vi "calibration setting.vi"() -> ()   [LabVIEW 2019, in "Calibration Lib.lvlib"]
uses:
  Calibration Lib.lvlib
  database.lvlib
panel:
  in  "Close":bool
  in  "Method 2 Verify":bool
  out "Error out":errorcluster
  in  "Calibration File Path":path
  out "Calibration String":string
  in  "Calibration Method":enum32{"Method 1", "Method 2"}(radio)=enum."Method 2"
  in  "Thresholds":bool
  in  "Method 2 Calibration":bool
  in  "Method 1 Calibration":bool
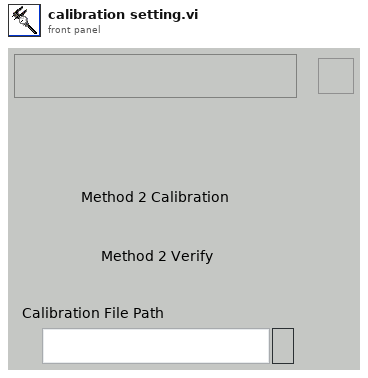
[diagram p1: front panel]
types:
  T1 = cluster{"Calibration Method":enum32{"Method 1", "Method 2"}, "Calibration File Path":path}
  T2 = enum8{"Enabled", "Disabled", "Disabled and Grayed Out"}
  T3 = cluster{"Calibration Method":u32, "Calibration File Path":path}[]
  T4 = cluster{"Calibration Method":u32, "Calibration File Path":path}
  T5 = cluster{"Calibration Method":enum32{"Method 1", "Method 2"}, string}
  T6 = cluster{i32, "date/time string":string, "date/time string":string, "table":string}
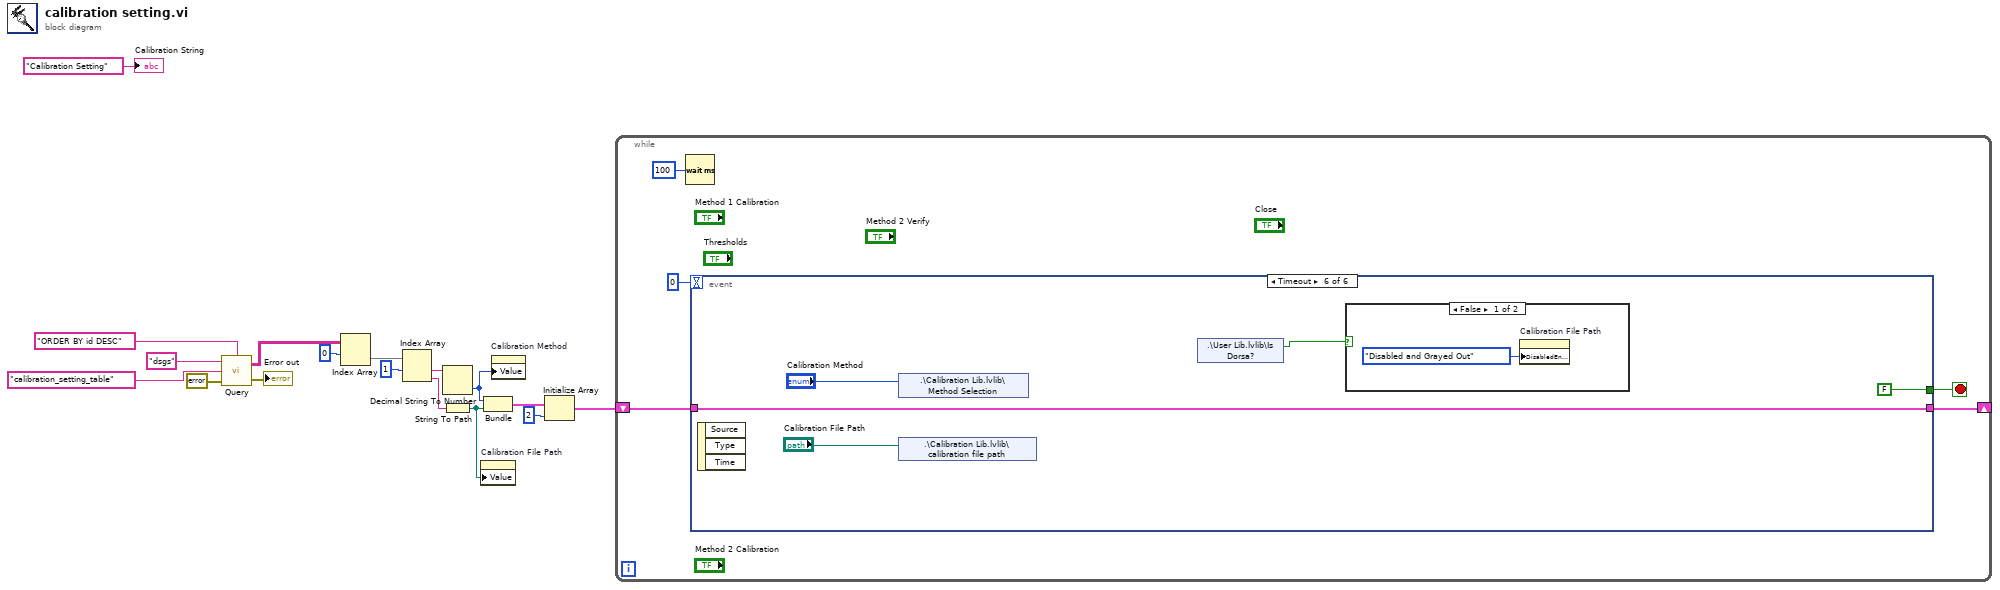
[diagram p0: block diagram]
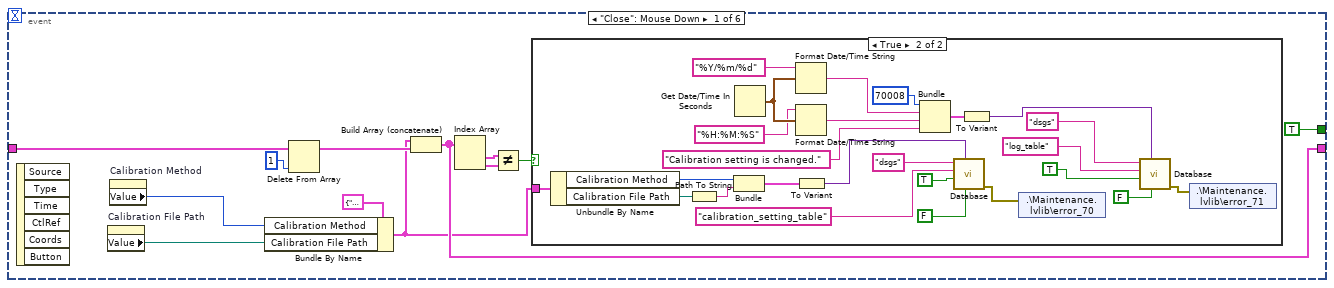
[diagram p2: hidden frame]
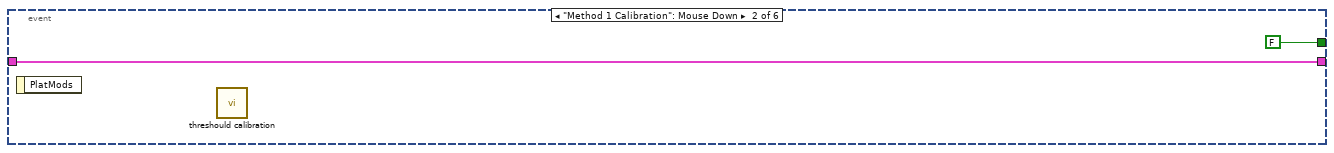
[diagram p4: hidden frame]
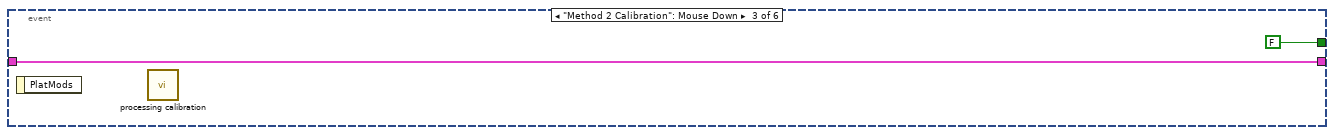
[diagram p5: hidden frame]
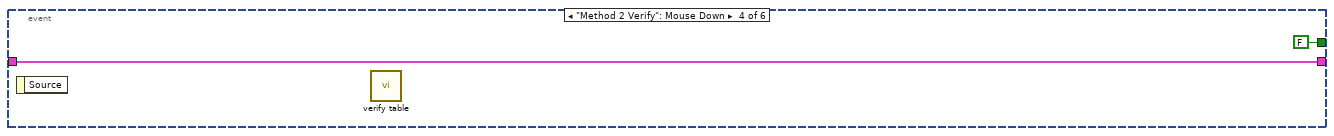
[diagram p6: hidden frame]
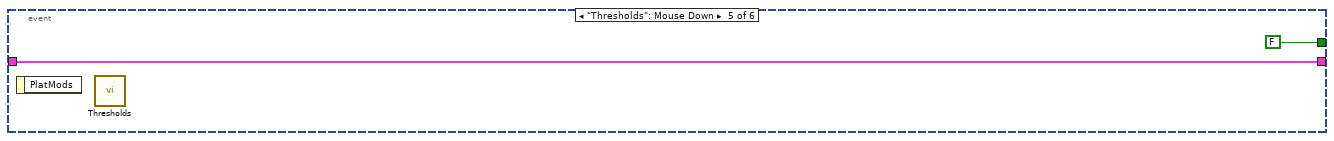
[diagram p7: hidden frame]
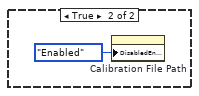
[diagram p8: hidden frame]
diagram:
  n1 = call "Query.vi"("Condition"="ORDER BY id DESC", "Error in"=errorcluster {"status"=FALSE, "code"=0, "source"=""}, "Table Name"="calibration_setting_table", "Connection Name"="dsgs") -> ("Error out"=→"Error out":errorcluster, "data"=w10:string[][])
  n2 = Index Array(array=w10, index (row)=0) -> (element=w8:string[])  [unwired: 1 in]
  n3 = Index Array(array=w8, index #1=1 ("index")) -> (element #1=w6:string, element #2=w4:string)  [unwired: 1 in]
  n4 = Decimal String To Number(string=w6) -> (number=w3:i32)  [unwired: 2 in, 1 out]
  n5 = String To Path(string=w4) -> (path=w2:path)
  n6 = property on="Calibration File Path" class="Path"("Value"=w2) -> ()  [unwired: 2 in, 2 out]
  n7 = Bundle(w3, w2) -> (w1:cluster{i32, path})  [unwired: 1 in]
  n8 = property on="Calibration Method" class="RadioBtnsControl (strict)"("Value"=w3) -> ()  [unwired: 2 in, 2 out]
  n9 = Initialize Array(w1, 2 ("dimension size")) -> (w15:cluster{i32, path}[])
  n10 = while {
    shift-right: [w18] -> _
    shift-left: w15 -> [w19]
    stop <- w21 stop-if-true
    n11 = Wait (ms)(milliseconds to wait=u32 100) -> ()  [unwired: 1 out]
    n12 = event shown="[5] Timeout" {
      selector: _ -> [_ _ _ _ _ _]
      dyn-events: _ -> [_ _ _ _ _ _]
      timeout: 0 -> [_ _ _ _ _ _]
      tunnel: [TRUE FALSE FALSE FALSE FALSE FALSE] -> w21
      tunnel: w19 -> [w30 w60 w62 w65 w66 w69]
      tunnel: [w26 w60 w62 w65 w66 w69] -> w18
      event "Close": Mouse Down {
        n13 = event-data() -> ()  [unwired: 1 in, 6 out]
        n14 = property on="Calibration File Path" class="Path"() -> ("Value"=w33:path)  [unwired: 2 in, 2 out]
        n15 = property on="Calibration Method" class="RadioBtnsControl (strict)"() -> ("Value"=w32:enum32{"Method 1", "Method 2"})  [unwired: 2 in, 2 out]
        n16 = Bundle By Name(cluster=T1 {"Calibration Method"=enum."Method 2", "Calibration File Path"=path ""}, "Calibration Method"=w32, "Calibration File Path"=w33) -> (w23:T1)
        n17 = Delete From Array(array=w30, index=1) -> (array with subset deleted=w28:T3)  [unwired: 1 in, 1 out]
        n18 = Build Array (concatenate)(w23, w28) -> (w26:T3)
        n19 = Index Array(array=w26) -> (element #1=w25:T4, element #2=w24:T4)  [unwired: 2 in]
        n20 = Not Equal?(x=w25, y=w24) -> (x != y?=w27:bool)
        n21 = case shown="True" w27 {
          tunnel: w23 -> [_ w39]
          frame False {
          }
          frame True {
            n22 = Unbundle By Name(w39) -> ("Calibration Method"=w37:enum32{"Method 1", "Method 2"}, "Calibration File Path"=w38:path)
            n23 = Path To String(path=w38) -> (string=w41:string)
            n24 = Bundle("Calibration Method"=w37, w41) -> (w40:T5)  [unwired: 1 in]
            n25 = Get Date/Time In Seconds() -> (seconds since 1Jan1904=w55:timestamp)
            n26 = Format Date/Time String(time format string (%c)="%Y/%m/%d", seconds (now)=w55) -> (date/time string=w56:string)  [unwired: 1 in]
            n27 = Format Date/Time String(time format string (%c)="%H:%M:%S", seconds (now)=w55) -> (date/time string=w57:string)  [unwired: 1 in]
            n28 = To Variant(anything=w40) -> (Variant=w42:variant)
            n29 = Bundle(70008, "date/time string"=w56, "date/time string"=w57, "table"="Calibration setting is changed.") -> (w58:T6)  [unwired: 1 in]
            n30 = call "Database.vi"("Delete row?"=FALSE, "Data"=w42, "Auto Increment ID?"=TRUE, "Table"="calibration_setting_table", "Connection"="dsgs") -> ("Error out"=w35:errorcluster)  [unwired: 6 in]
            n31 = To Variant(anything=w58) -> (Variant=w59:variant)
            n32 = shared-variable ".\\Maintenance.lvlib\\error_70"(w35) -> ()  [unwired: 1 in, 1 out]
            n33 = call "Database.vi"("Delete row?"=FALSE, "Data"=w59, "Auto Increment ID?"=TRUE, "Table"="log_table" ("table"), "Connection"="dsgs" ("table")) -> ("Error out"=w36:errorcluster)  [unwired: 6 in]
            n34 = shared-variable ".\\Maintenance.lvlib\\error_71"(w36) -> ()  [unwired: 1 in, 1 out]
          }
        }
      }
      event "Method 1 Calibration": Mouse Down {
        n35 = event-data() -> ()  [unwired: 1 in, 1 out]
        n36 = call "threshould calibration.vi"() -> ()  [unwired: 12 in]
      }
      event "Method 2 Calibration": Mouse Down {
        n37 = event-data() -> ()  [unwired: 1 in, 1 out]
        n38 = call "processing calibration.vi"() -> ()  [unwired: 12 in]
      }
      event "Method 2 Verify": Mouse Down {
        n39 = event-data() -> ()  [unwired: 1 in, 1 out]
        n40 = call "verify table.vi"() -> ()  [unwired: 12 in]
      }
      event "Thresholds": Mouse Down {
        n41 = event-data() -> ()  [unwired: 1 in, 1 out]
        n42 = call "Thresholds.vi"() -> ()  [unwired: 12 in]
      }
      event Timeout {
        n43 = event-data() -> ()  [unwired: 1 in, 3 out]
        n44 = shared-variable ".\\Calibration Lib.lvlib\\Method Selection"("Calibration Method") -> ()  [unwired: 1 in, 1 out]
        n45 = shared-variable ".\\Calibration Lib.lvlib\\calibration file path"("Calibration File Path") -> ()  [unwired: 1 in, 1 out]
        n46 = shared-variable ".\\User Lib.lvlib\\Is Dorsa?"() -> (w68:bool)  [unwired: 1 in, 1 out]
        n47 = case shown="False" w68 {
          frame False {
            n48 = property on="Calibration File Path" class="Path"("DisabledEnum"=T2."Disabled and Grayed Out" ("Disabled")) -> ()  [unwired: 2 in, 2 out]
          }
          frame True {
            n49 = property on="Calibration File Path" class="Path"("DisabledEnum"=T2."Enabled" ("Disabled")) -> ()  [unwired: 2 in, 2 out]
          }
        }
      }
    }
  }
  "Calibration String" <- "Calibration Setting" ("Calibration String")
